vi "Read Name.vi"(3 "((Pointer))":refnum<class "_Pointer.lvclass">) -> (1 "Name Out":string)   [LabVIEW 2024, in "_Pointer.lvclass"]
uses:
  _Pointer.lvclass
  _Pointer.lvclass/_Pointer.ctl
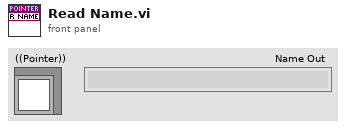
[diagram p1: front panel]
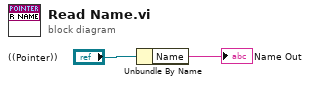
[diagram p0: block diagram]
diagram:
  n1 = Unbundle By Name("((Pointer))") -> ("Name"=→"Name Out":string)
